vi "centre_front_panel.vi"(11 "VI in":refnum<vi>) -> ()   [LabVIEW 2023]
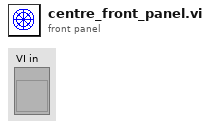
[diagram p1: front panel]
types:
  T1 = typedef "LVPointTypeDef.ctl" = cluster{"Horizontal":i16, "Vertical":i16}
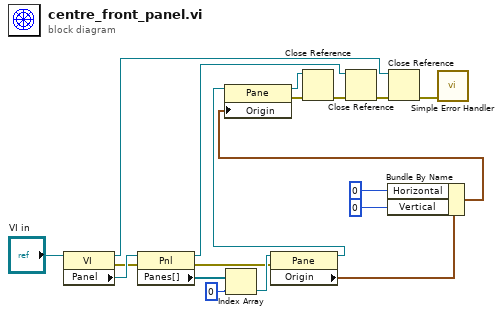
[diagram p0: block diagram]
diagram:
  n1 = property class="VI"(reference="VI in") -> (reference out=w19:refnum<vi>, error out=w2:errorcluster, "Panel"=w3:refnum<vi>)  [unwired: 1 in]
  n2 = property class="Pnl"(reference=w3, error in=w2) -> (reference out=w18:refnum<vi>, error out=w4:errorcluster, "Panes[]"=w5:refnum<vi>[])
  n3 = Index Array(array=w5, index=0) -> (element=w7:refnum<vi>)
  n4 = property class="Pane"(reference=w7, error in=w4) -> (reference out=w15:refnum<vi>, "Origin"=w16:T1)  [unwired: 1 out]
  n5 = Bundle By Name(cluster=w16, "Horizontal"=i16 0, "Vertical"=i16 0) -> (w17:T1)
  n6 = property class="Pane"(reference=w15, "Origin"=w17) -> (reference out=w11:refnum<vi>, error out=w10:errorcluster)  [unwired: 1 in]
  n7 = Close Reference(reference=w11, error in (no error)=w10) -> (error out=w12:errorcluster)
  n8 = Close Reference(reference=w18, error in (no error)=w12) -> (error out=w13:errorcluster)
  n9 = Close Reference(reference=w19, error in (no error)=w13) -> (error out=w14:errorcluster)
  n10 = call <vilib>:"Simple Error Handler.vi"("error in (no error)"=w14) -> ()  [unwired: 4 in, 5 out]
